vi "Assert Equal_Value_Variant.vi"(5 "Assert Only? (F)":bool, 6 "error code (1)":i32=1, 7 "Label":string, 8 "error in (no error)":errorcluster, 10 "Y":variant, 11 "X":variant) -> (0 "error out":errorcluster)   [LabVIEW 2009, in "Caraya.lvlib" / "Assert.lvclass"]
doc: "Generates an error if the input condition is not met.\n\n--\nCopyright © 2015 JKI All rights reserved.\n\nAuthor: Tomi Maila <tomi.maila@jki.net>\n\nThis library is provided \"AS IS\" ,WITHOUT WARRANTIES OR\nCONDITIONS OF ANY KIND, either express or implied.\n\nJKI -- jki.net"
uses:
  Assert.lvclass
  <vilib>/Utility/VariantDataType/VariantType.lvlib
panel:
  # "Copyright © 2015 JKI All rights reserved.\n\nAuthor: Tomi Maila <tomi.maila@jki.net>\n\nThis library is provided \"AS IS\" ,WITHOUT WARRANTIES OR\nCONDITIONS OF ANY KIND, either express or implied.\n\nJKI -- jki.net"
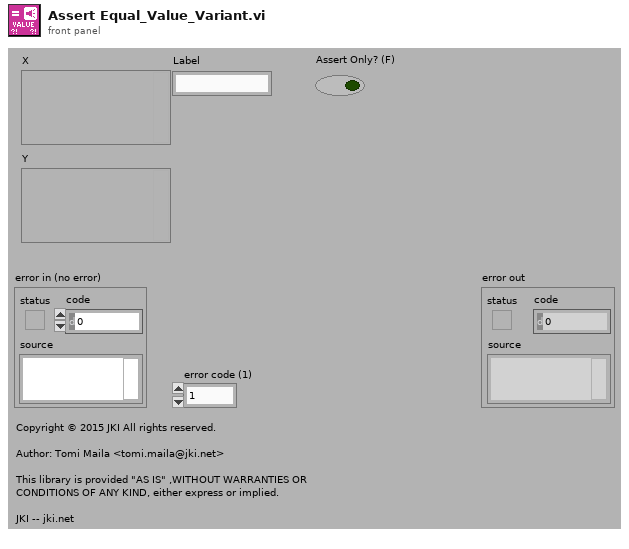
[diagram p1: front panel]
types:
  T1 = typedef "VariantType.lvlib/Type.ctl" = enum8{"Invalid Type", "Void", "I8", "I16", "I32", "I64", "U8", "U16", "U32", "U64", "Single Float", "Double Float", "Extended Float", "Single Complex", "Double Complex", "Extended Complex", "Enum U8", "Enum U16", "Enum U32", "Enum U64", "Single Float With Unit", "Double Float With Unit", "Extended Float With Unit", "Single Complex with Unit", "Double Complex with Unit", "Extended Complex with Unit", "Boolean", "String", "Path", "Picture", "Tag", "Array", "Cluster", "Variant", "LV Variant", "Waveform", "Timestamp", "Digital Waveform", "Digital Data", "ExpressData", "Refnum", "External Data", "VI", "Poly VI", "LabVIEW Class Instance", "Fixed Point"}
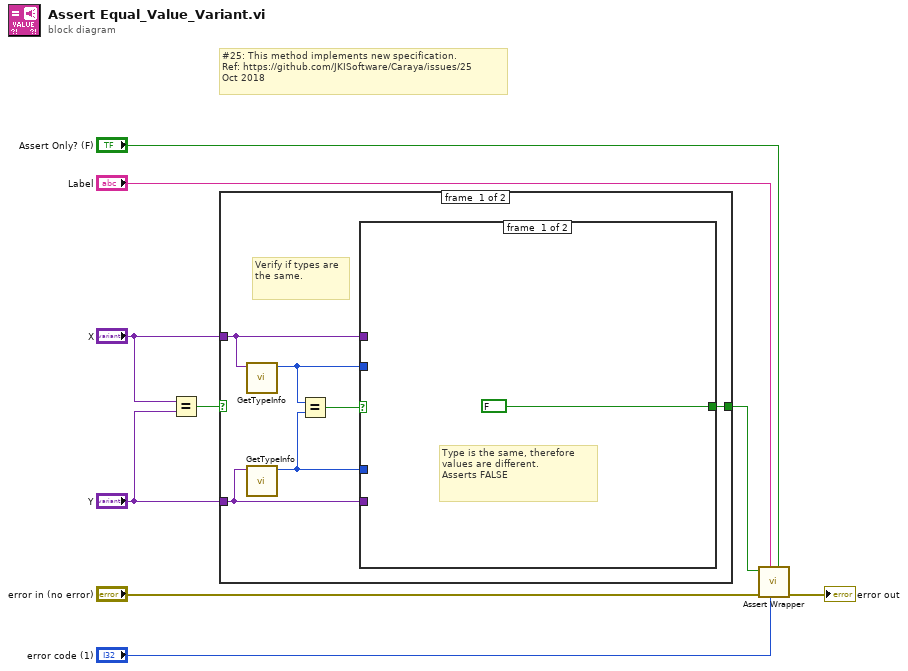
[diagram p0: block diagram]
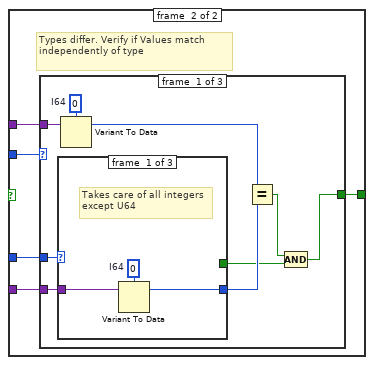
[diagram p2: hidden frame]
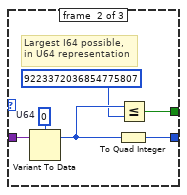
[diagram p3: hidden frame]
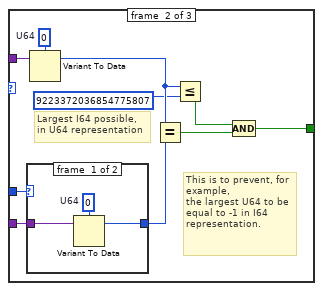
[diagram p5: hidden frame]
diagram:
  # "#25: This method implements new specification.\nRef: https://github.com/JKISoftware/Caraya/issues/25\nOct 2018"
  n1 = Equal?(x="X", y="Y") -> (x = y?=w4:bool)
  n2 = case shown="False" w4 {
    selector: w4 -> [_ w53]
    tunnel: "X" -> [w15 _]
    tunnel: [w13 w53] -> w2
    tunnel: "Y" -> [w14 _]
    frame #0 {
      # "Verify if types are the same."
      n3 = call <vilib>:"GetTypeInfo.vi"("Variant"=w15) -> ("Type Enum"=w11:T1)  [unwired: 6 in, 4 out]
      n4 = call <vilib>:"GetTypeInfo.vi"("Variant"=w14) -> ("Type Enum"=w10:T1)  [unwired: 6 in, 4 out]
      n5 = Equal?(x=w11, y=w10) -> (x = y?=w12:bool)
      n6 = case shown="False" w12 {
        tunnel: w15 -> [_ w20]
        tunnel: w14 -> [_ w19]
        tunnel: [FALSE w17] -> w13
        tunnel: w11 -> [_ w21]
        tunnel: w10 -> [_ w18]
        frame #0 {
          # "Type is the same, therefore values are different.\nAsserts FALSE"
        }
        frame #1 {
          # "Types differ. Verify if Values match independently of type"
          n7 = case shown="\"I8\"..\"U32\", \"Enum U8\"..\"Enum U32\"" w21 {
            tunnel: w20 -> [w29 w48 _]
            tunnel: w19 -> [w28 w47 _]
            tunnel: w18 -> [w27 w46 _]
            tunnel: [w22 w40 _] -> w17
            frame #0 {
              w30 = i64 0  # I64
              n8 = case shown="\"U64\"" w27 {
                tunnel: w28 -> [w32 w38 _]
                tunnel: [w31 w35 _] -> w25
                tunnel: [_ w34 _] -> w24
                frame #0 {
                  w33 = i64 0  # I64
                  # "Takes care of all integers\nexcept U64"
                  n9 = Variant To Data(Variant=w32, type=w33) -> (data=w31:i64)  [unwired: 1 in, 1 out]
                }
                frame #1 {
                  w39 = u64 0  # U64
                  # "Largest I64 possible,\nin U64 representation"
                  n10 = Variant To Data(Variant=w38, type=w39) -> (data=w37:u64)  [unwired: 1 in, 1 out]
                  n11 = To Quad Integer(1:w37) -> (0:w35:i64)
                  n12 = Less Or Equal?(x=w37, y=u64 9223372036854775807) -> (x <= y?=w34:bool)
                }
                frame #2 {
                }
              }
              n13 = Variant To Data(Variant=w29, type=w30) -> (data=w26:i64)  [unwired: 1 in, 1 out]
              n14 = Equal?(x=w26, y=w25) -> (x = y?=w23:bool)
              n15 = Compound Arithmetic op=AND(w23, w24) -> (w22:bool)
            }
            frame #1 {
              w49 = u64 0  # U64
              # "This is to prevent, for example, \nthe largest U64 to be equal to -1 in I64 representation."
              # "Largest I64 possible,\nin U64 representation"
              n16 = case shown="\"I8\"..\"U32\", \"Enum U8\"..\"Enum U32\"" w46 {
                tunnel: w47 -> [w51 _]
                tunnel: [w50 _] -> w45
                frame #0 {
                  w52 = u64 0  # U64
                  n17 = Variant To Data(Variant=w51, type=w52) -> (data=w50:u64)  [unwired: 1 in, 1 out]
                }
                frame #1 {
                }
              }
              n18 = Variant To Data(Variant=w48, type=w49) -> (data=w44:u64)  [unwired: 1 in, 1 out]
              n19 = Equal?(x=w44, y=w45) -> (x = y?=w41:bool)
              n20 = Less Or Equal?(x=w44, y=u64 9223372036854775807) -> (x <= y?=w42:bool)
              n21 = Compound Arithmetic op=AND(w42, w41) -> (w40:bool)
            }
            frame #2 {
              # "All non-integer representations must be of same type to potentially assert True"
            }
          }
        }
      }
    }
    frame #1 {
      # "If both Value and Type match, asserts TRUE"
    }
  }
  n22 = call "Assert Wrapper.vi"("Assert Only? (F)"="Assert Only? (F)", "error code (1)"="error code (1)", "Label"="Label", "error in (no error)"="error in (no error)", "Assert?"=w2) -> ("error out"=→"error out":errorcluster)  [unwired: 6 in]
